vi "Assert String Not Contains String.vi"(5 "Needle":string, 7 "Message (\"\")":string, 8 "error in (no error)":errorcluster, 10 "Haystack":string) -> (0 "error out":errorcluster)   [LabVIEW 2017, in "Assertion.lvlib"]
doc: "Asserts that <B>haystack</B> does not contain <B>needle</B>. Does nothing if an error occurred before this node runs. Returns an error if the assertion failed. Optionally adds a message to the error message if the assertion failed."
uses:
  Assertion.lvlib
  Constraint/LogicalNot/LogicalNot.lvclass
  Constraint/StringContains/StringContains.lvclass
  C:/Users/de200256/Code/logmanoriginal/lvunit/Constraint/Constraint/Constraint.lvclass
  Constraint/UnaryOperator/UnaryOperator.lvclass
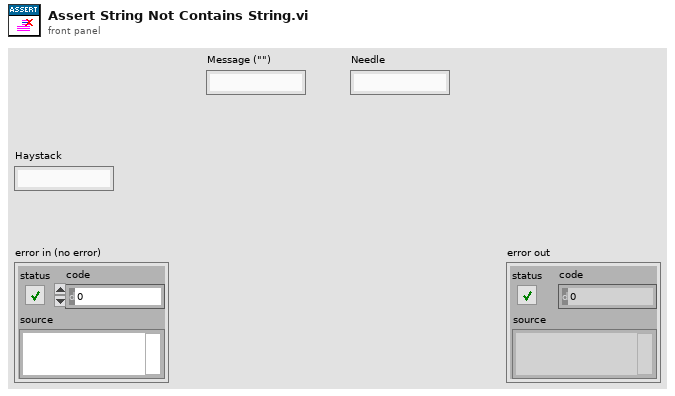
[diagram p1: front panel]
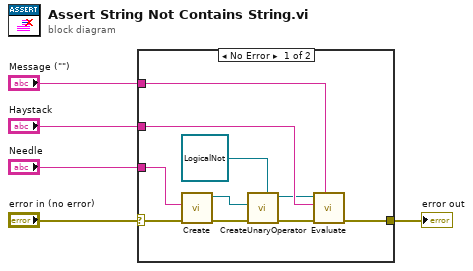
[diagram p0: block diagram]
diagram:
  n1 = case shown="No Error" "error in (no error)" {
    selector: "error in (no error)" -> [w11 w16]
    tunnel: "Haystack" -> [w14 _]
    tunnel: [w13 w16] -> w4
    tunnel: "Message (\"\")" -> [w12 _]
    tunnel: "Needle" -> [w10 _]
    frame No Error {
      n2 = call "Create.vi"("error in (no error)"=w11, "Needle"=w10) -> ("error out"=w15:errorcluster, "StringContains"=w7:refnum<class "StringContains.lvclass">)  [unwired: 8 in]
      n3 = call-dynamic "CreateUnaryOperator.vi"("UnaryOperator In"=refnum<class "LogicalNot.lvclass"> refnum ("Constraint.lvlib:LogicalNot.lvclass"), "error in (no error)"=w15, "Constraint"=w7) -> ("error out"=w9:errorcluster, "UnaryOperator"=w6:refnum<class "UnaryOperator.lvclass">)  [unwired: 7 in]
      n4 = call-dynamic "Evaluate.vi"("Message (\"\")"=w12, "error in (no error)"=w9, "Actual"=w14, "Constraint in"=w6) -> ("error out"=w13:errorcluster)  [unwired: 6 in, 1 out]
    }
    frame Error {
    }
  }
  "error out" <- w4
